vi "LaneExtractorHenesUseNetwork.vi"() -> ()   [LabVIEW 2024]
uses:
  <vilib>/userDefined/High Color/IMAQdx.ctl
  System.Windows.Forms
  <vilib>/Instr/_visa.llb/VISA Set IO Buffer Mask.ctl
  <vilib>/Instr/_visa.llb/VISA Flush IO Buffer Mask.ctl
  <vilib>/Instr/_visa.llb/VISA Configure Serial Port (Instr).vi
  <vilib>/vision/driver/NI_Vision_Acquisition_Software.lvlib
panel:
  in  "Current_image":refnum<k24>(container)
  in  "Right_lane":refnum<k24>(container)
  in  "Left_lane":refnum<k24>(container)
  out "error out 5":errorcluster
  out "inference time":string="imagedecode_time: 0 ms, inference_time: 10 ms, image_save_time: 0 ms, lane_determine_time: 4 ms, debug_image_save_time: 2 ms, calculation_time: 2 ms, stanley_time: 0 ms, debug_image2_save_time: 6 ms, both"
  out "error out 3":errorcluster
  out "Image_String":string
  in  "File Path":path=path "C:/Users/JungiHong/OneDrive/Hongik/HI-RACE/2026-01/platform_1_5/ExperimentModules/LaneTracking/forTrainImages/frame_014.jpg"
  in  "UseVideo":bool
  in  "Cam No.":T1="cam0"
  in  "input_spd":i16
  in  "HENES":refnum<visa-resource-name>="COM5"
  out "E-STOP":bool
  out "Remote_M/A":bool
  out "Steer_Feed":dbl
  out "Alive_PCU":u8(slide) scale=0.0..254.0
  out "Gear_Feed":u8
  out "Speed_Feed(RPM)":dbl format="%#_g rpm"
  out "버퍼 읽기":string
  out "Speed_Feed(m/s)":dbl
  in  "HLV_Gear":u8
  in  "HLV_A/M":bool=TRUE
  in  "HLV_E-stop":bool
  out "HENES Loop Time":u32=20
  in  "v(Velocity)m/s":dbl=1.0
  in  "k(Gain)":dbl=1.0
  out "δ(OutputSteer)degrees":dbl=3.398135469980901
  out "changearray":u32=4
  out "CV Loop Time":u32=103
  in  "stop":bool
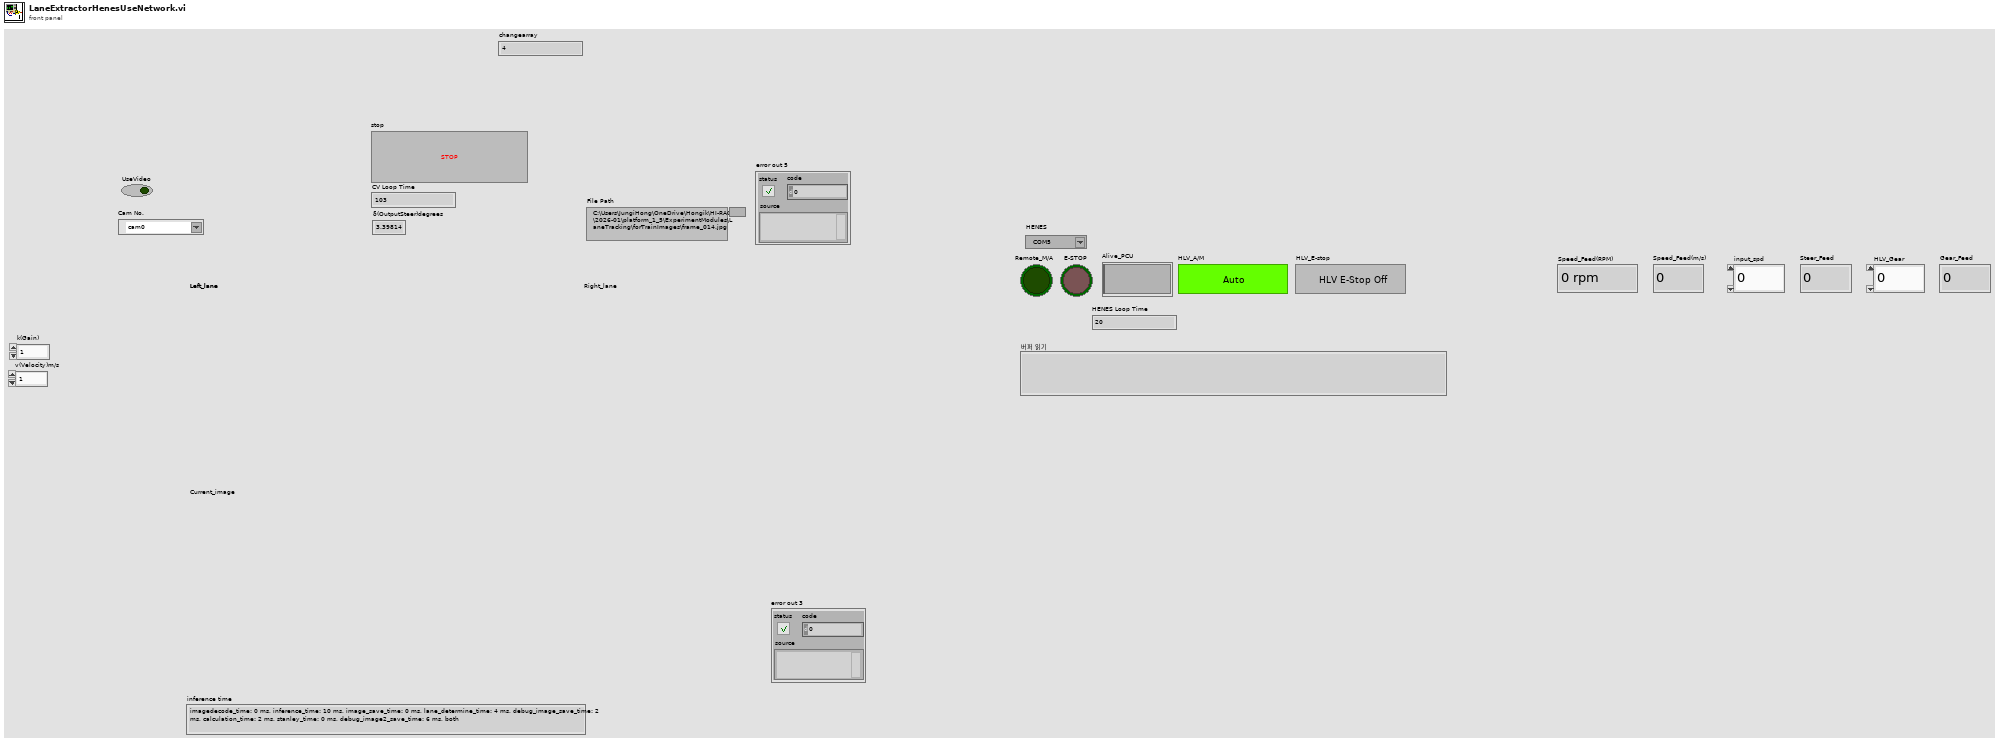
[diagram p1: front panel]
types:
  T1 = typedef "IMAQdx.ctl" = refnum<k21>
  T2 = cluster{"HENES_M/A":u8, "HENES_E-Stop":u8, "HENES_Gear":u8, "HENES_Speed":i16, "HENES_Steer":i16, "HENES_Alive":u8}
  T3 = typedef "VISA Flush IO Buffer Mask.ctl" = u16
  T4 = typedef "VISA Set IO Buffer Mask.ctl" = u16
  T5 = cluster{"HLV_M/A_Status":u8, "HLV_E-Stop":u8, "HLV_Gear":u8, "HLV_Speed":i16, "HLV_Steer":i16, "HLV_Alive":u8}
  T6 = typedef "IMAQ Image.ctl" = refnum<image>
  T7 = cluster{"Global Rectangle":i32[], "Contours":cluster{"ID":enum32{"External", "Internal"}, "Type":u32, "Coordinates":i32[]}[]}
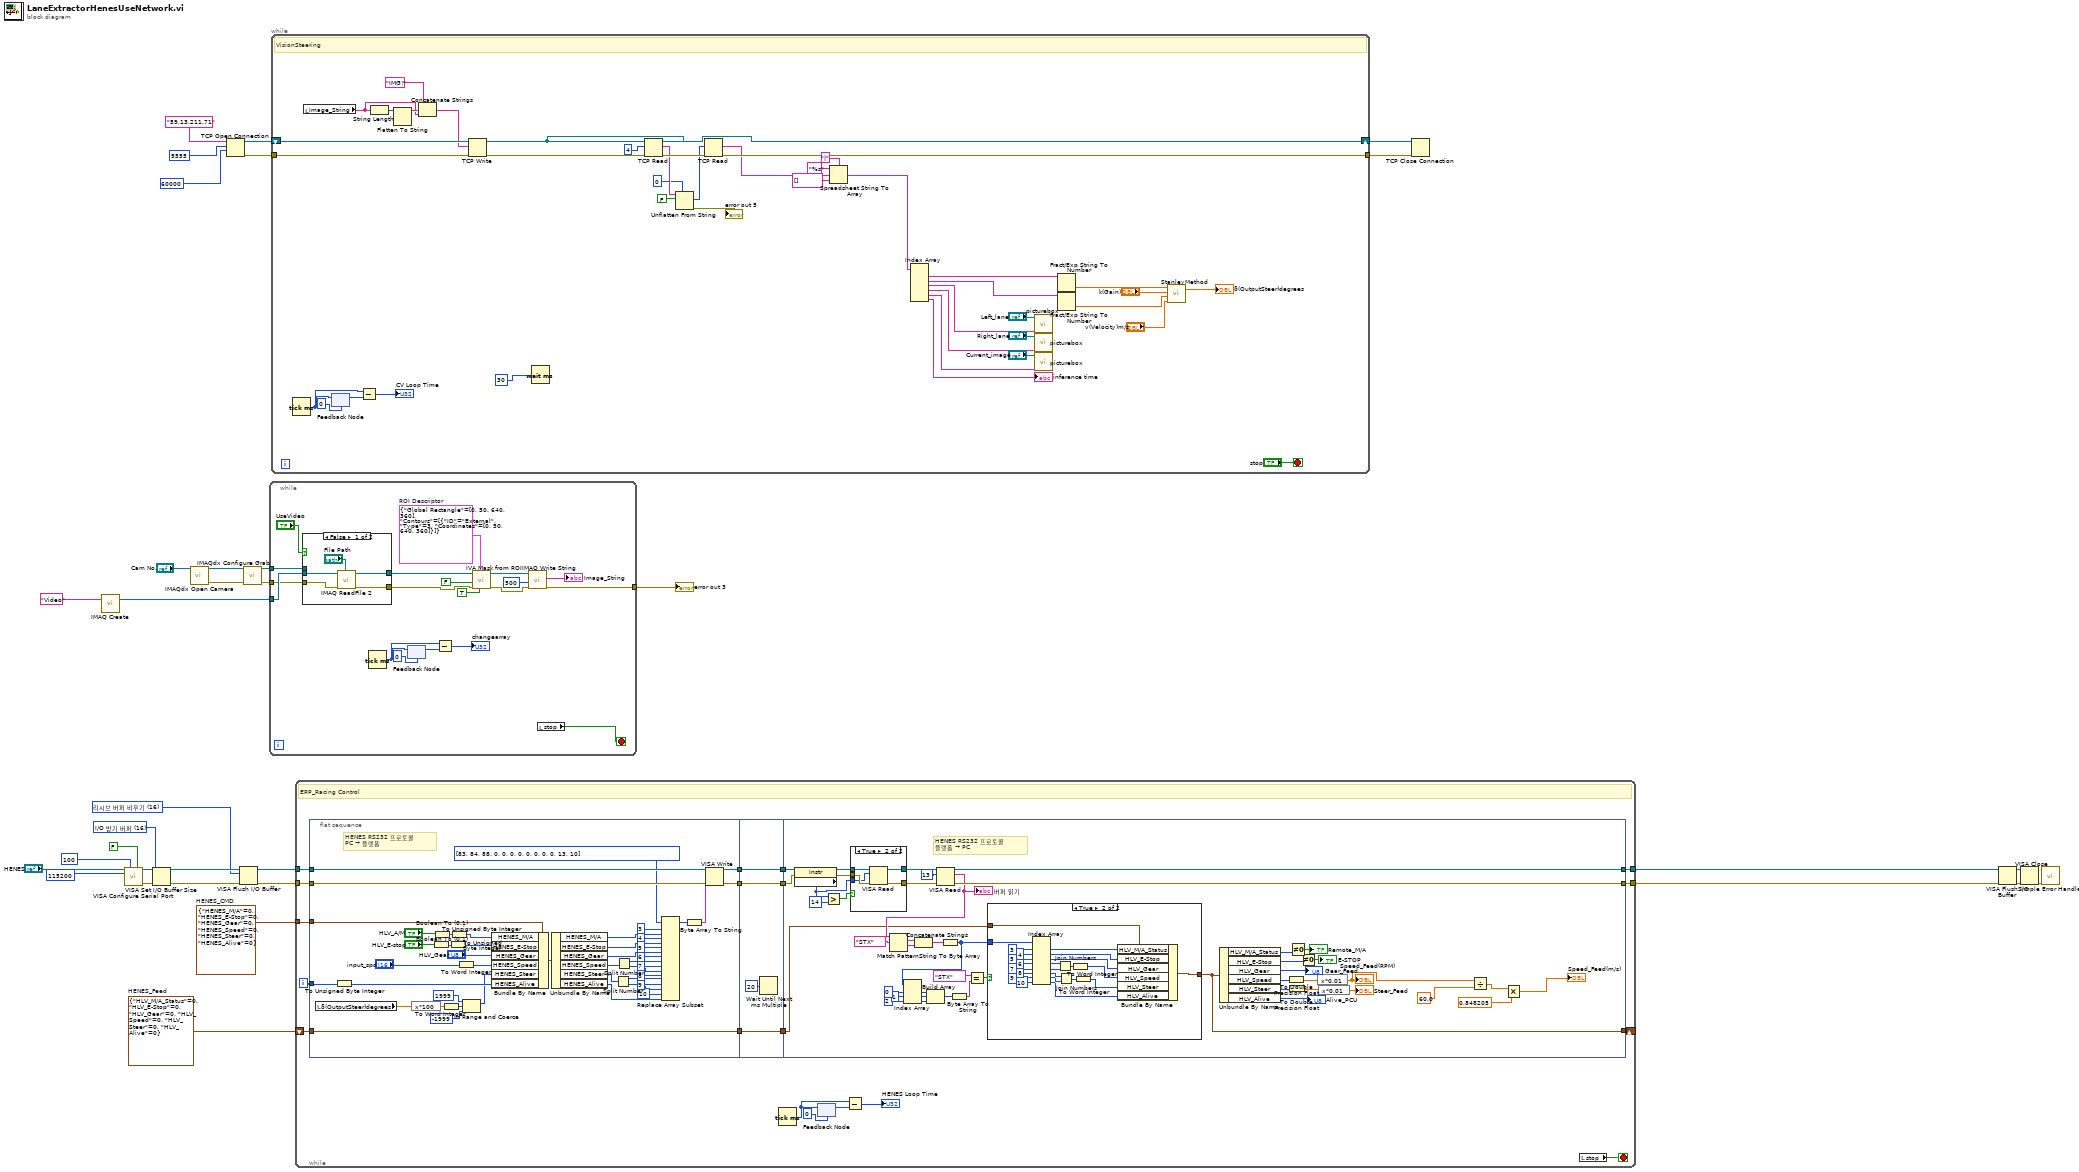
[diagram p0: block diagram]
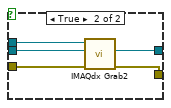
[diagram p4: hidden frame]
diagram:
  w15 = T2 {"HENES_M/A"=0, "HENES_E-Stop"=0, "HENES_Gear"=0, "HENES_Speed"=0, "HENES_Steer"=0, "HENES_Alive"=0}  # HENES_CMD
  w18 = T3 16 items=["리시브 버퍼 비우기"=16, "전달 버퍼 디바이스에 쓰기"=32, "리시브 버퍼 비우기(I/O 없음)"=64, "전달 버퍼 비우기"=128] ("Mask")
  w21 = T4 16 items=["I/O 받기 버퍼"=16, "I/O 전달 버퍼"=32, "I/O 받기와 전달 버퍼"=48] ("Mask")
  w25 = T5 {"HLV_M/A_Status"=0, "HLV_E-Stop"=0, "HLV_Gear"=0, "HLV_Speed"=0, "HLV_Steer"=0, "HLV_Alive"=0}  # HENES_Feed
  n1 = call "IMAQ Create"("Image Name"="Video") -> ("New Image"=w33:T6)  [unwired: 4 in, 1 out]
  n2 = call-poly "VISA Configure Serial Port"("VISA resource name"="HENES", "timeout (10sec)"=u32 100, "Enable Termination\nChar (T)"=FALSE ("Enable Termination\nChar (T)"), "baud rate (9600)"=u32 115200) -> ("VISA resource name out"=w17:refnum<visa-resource-name>, "error out"=w16:errorcluster)  [unwired: 10 in]
  n3 = VISA Set I/O Buffer Size(VISA resource name=w17, mask (16)=w21, error in (no error)=w16) -> (VISA resource name out=w20:refnum<visa-resource-name>, error out=w19:errorcluster)  [unwired: 1 in]
  n4 = call <vilib>:"IMAQdx Open Camera.vi"("Session In"="Cam No.") -> ("error out"=w11:errorcluster, "Session Out"=w12:T1)  [unwired: 9 in]
  n5 = TCP Open Connection(address="59.13.211.71", remote port or service name=u16 5555, timeout ms (60000)=60000) -> (connection ID=w3:refnum<k5>, error out=w4:errorcluster)  [unwired: 2 in]
  n6 = VISA Flush I/O Buffer(VISA resource name=w20, mask (16)=w18, error in (no error)=w19) -> (VISA resource name out=w30:refnum<visa-resource-name>, error out=w29:errorcluster)
  n7 = call <vilib>:"IMAQdx Configure Grab.vi"("error in"=w11, "Session In"=w12) -> ("error out"=w10:errorcluster, "Session Out"=w13:T1)  [unwired: 8 in]
  n8 = while {
    tunnel: w33 -> [w48]
    tunnel: w13 -> [w47]
    tunnel: w10 -> [w46]
    tunnel: [w38] -> w8
    stop <- w53 stop-if-true
    w43 = T7 {"Global Rectangle"=[0, 50, 640, 360], "Contours"=[{"ID"=enum."External", "Type"=3, "Coordinates"=[0, 50, 640, 360]}]}  # ROI Descriptor
    n9 = case shown="False" "UseVideo" {
      tunnel: w48 -> [w56 w63]
      tunnel: [w58 w62] -> w36
      tunnel: [w57 w61] -> w41
      tunnel: w47 -> [_ w60]
      tunnel: w46 -> [w54 w59]
      frame False {
        n10 = call "IMAQ ReadFile 2"("File Path"="File Path", "error in (no error)"=w54, "Image"=w56) -> ("error out"=w58:errorcluster, "Image Out"=w57:T6)  [unwired: 4 in, 3 out]
      }
      frame True {
        n11 = call <vilib>:"IMAQdx Grab2.vi"("error in"=w59, "Image In"=w63, "Session In"=w60) -> ("error out"=w62:errorcluster, "Image Out"=w61:T6)  [unwired: 5 in, 2 out]
      }
    }
    n12 = Tick Count (ms)() -> (millisecond timer value=w49:u32)
    n13 = feedback #1(u32 0 ("millisecond timer value")) -> (w50:u32)
    n14 = feedback-in #1(w49) -> ()
    n15 = Subtract(x=w49, y=w50) -> (x-y=→"changearray":u32)
    n16 = call <vilib>:"IVA Mask from ROI.vi"("Shrink"=TRUE, "ROI Descriptor"=w43, "error in (no error)"=w36, "Out / In"=FALSE, "Image Src"=w41) -> ("error out"=w35:errorcluster, "Image Out"=w39:T6)  [unwired: 5 out]
    n17 = call-poly "IMAQ Write String"("error in (no error)"=w35, "Image Quality"=u32 500, "Image"=w39) -> ("error out"=w38:errorcluster, "FileString"=→"Image_String":string)  [unwired: 6 in, 1 out]
    n18 = local read "stop"() -> (w53:bool)
  }
  "error out 3" <- w8
  n19 = while {
    tunnel: w4 -> [w77]
    tunnel: [w89] -> w2
    shift-right: [w87] -> w1
    shift-left: w3 -> [w78]
    stop <- "stop" stop-if-true
    # "VisionSteering"
    n20 = Tick Count (ms)() -> (millisecond timer value=w105:u32)
    n21 = local read "Image_String"() -> (w72:string)
    n22 = feedback #2(u32 0 ("millisecond timer value")) -> (w104:u32)
    n23 = feedback-in #2(w105) -> ()
    n24 = Subtract(x=w105, y=w104) -> (x-y=→"CV Loop Time":u32)
    n25 = String Length(string=w72) -> (length=w74:i32)
    n26 = Flatten To String(anything=w74) -> (data string=w73:string)  [unwired: 3 in, 2 out]
    n27 = Concatenate Strings("IMG!" ("Image_String"), w73, w72) -> (w70:string)
    n28 = TCP Write(connection ID=w78, data in=w70, error in (no error)=w77) -> (connection ID out=w79:refnum<k5>, error out=w80:errorcluster)  [unwired: 1 in, 1 out]
    n29 = Wait (ms)(milliseconds to wait=u32 30) -> ()  [unwired: 1 out]
    n30 = TCP Read(connection ID=w79, bytes to read=4, error in (no error)=w80) -> (connection ID out=w87:refnum<k5>, data out=w84:string, error out=w86:errorcluster)  [unwired: 2 in]
    n31 = Unflatten From String(type=u32 0 ("CV Loop Time 2"), binary string=w84, data includes array or string size? (T)=FALSE) -> (value=w85:u32, error out=→"error out 5":errorcluster)  [unwired: 2 in, 1 out]
    n32 = TCP Read(connection ID=w79, bytes to read=w85, error in (no error)=w86) -> (data out=w88:string, error out=w89:errorcluster)  [unwired: 2 in, 1 out]
    n33 = Spreadsheet String To Array(delimiter (Tab)="|", format string="%s", spreadsheet string=w88, array type (2D Dbl)=string[] []) -> (array=w90:string[])
    n34 = Index Array(array=w90) -> (element #1=w93:string, element #2=w92:string, element #3=w69:string, element #4=w65:string, element #5=w64:string, element #6=→"inference time":string)  [unwired: 6 in]
    n35 = call "picturebox.vi"("s"=w69, "PictureBox"="Left_lane") -> ()  [unwired: 10 in]
    n36 = call "picturebox.vi"("s"=w65, "PictureBox"="Right_lane") -> ()  [unwired: 10 in]
    n37 = call "picturebox.vi"("s"=w64, "PictureBox"="Current_image") -> ()  [unwired: 10 in]
    n38 = Fract/Exp String To Number(string=w93) -> (number=w100:dbl)  [unwired: 3 in, 1 out]
    n39 = Fract/Exp String To Number(string=w92) -> (number=w99:dbl)  [unwired: 3 in, 1 out]
    n40 = call "StanleyMethod.vi"("v(Velocity)m/s"="v(Velocity)m/s", "e(Cross-Track Err)m/s"=w99, "k(Gain)"="k(Gain)", "ψ(Heading Err)radian"=w100) -> ("δ(OutputSteer)degrees"=→"δ(OutputSteer)degrees":dbl)  [unwired: 1 out]
  }
  n41 = while {
    tunnel: w30 -> [w125]
    tunnel: w29 -> [w124]
    tunnel: [w118] -> w28
    tunnel: [w117] -> w27
    shift-right: [w112] -> _
    shift-left: w25 -> [w115]
    tunnel: w15 -> [w113]
    i -> [w119]
    stop <- w107 stop-if-true
    # "ERP_Racing Control"
    n42 = flat-sequence {
      tunnel: [w168] -> w122
      tunnel: [w167] -> w120
      tunnel: w125 -> [w170]
      tunnel: w124 -> [w169]
      tunnel: w119 -> [w166]
      tunnel: [w165] -> w116
      tunnel: w115 -> [w165]
      tunnel: w113 -> [w164]
      tunnel: [w174] -> w123
      tunnel: w122 -> [w174]
      tunnel: [w173] -> w121
      tunnel: w120 -> [w173]
      tunnel: w116 -> [w171]
      tunnel: [w171] -> w114
      tunnel: w123 -> [w202]
      tunnel: w121 -> [w201]
      tunnel: [w219] -> w118
      tunnel: [w218] -> w117
      tunnel: w114 -> [w193]
      tunnel: [w191] -> w112
      frame #0 {
        # "HENES RS232 프로토콜\nPC → 플랫폼"
        n43 = local read "δ(OutputSteer)degrees"() -> (w126:dbl)
        n44 = To Unsigned Byte Integer(number=w166) -> (unsigned 8bit integer=w153:u8)
        n45 = expression code="x*100"(w126) -> (w128:dbl)
        n46 = Boolean To (0,1)(Boolean="HLV_E-stop") -> (0, 1=w148:i16)
        n47 = Boolean To (0,1)(Boolean="HLV_A/M") -> (0, 1=w149:i16)
        n48 = To Word Integer(number=w128) -> (16bit integer=w131:i16)
        n49 = To Unsigned Byte Integer(number=w148) -> (unsigned 8bit integer=w146:u8)
        n50 = To Unsigned Byte Integer(number=w149) -> (unsigned 8bit integer=w147:u8)
        n51 = To Word Integer(number="input_spd") -> (16bit integer=w140:i16)
        n52 = In Range and Coerce(upper limit=i16 1999 ("상위 리미트"), x=w131, lower limit=i16 -1999 ("상위 리미트")) -> (coerced(x)=w139:i16)  [unwired: 1 out]
        n53 = Bundle By Name(cluster=w164, "HENES_M/A"=w147, "HENES_E-Stop"=w146, "HENES_Gear"="HLV_Gear", "HENES_Speed"=w140, "HENES_Steer"=w139, "HENES_Alive"=w153) -> (w157:T2)
        n54 = Unbundle By Name(w157) -> ("HENES_M/A"=w143:u8, "HENES_E-Stop"=w142:u8, "HENES_Gear"=w132:u8, "HENES_Speed"=w135:i16, "HENES_Steer"=w138:i16, "HENES_Alive"=w152:u8)
        n55 = Split Number(x=w138) -> (hi(x)=w137:u8, lo(x)=w136:u8)
        n56 = Split Number(x=w135) -> (hi(x)=w134:u8, lo(x)=w133:u8)
        n57 = Replace Array Subset(array=u8[] [83, 84, 88, 0, 0, 0, 0, 0, 0, 0, 0, 13, 10] ("unsigned byte array"), new element #1=w143, index #1=3, new element #2=w142, index #2=4, new element #3=w132, index #3=5, new element #4=w134, index #4=6, new element #5=w133, index #5=7, new element #6=w137, index #6=8, new element #7=w136, index #7=9, new element #8=w152, index #8=10) -> (w155:u8[])
        n58 = Byte Array To String(unsigned byte array=w155) -> (string=w154:string)
        n59 = VISA Write(VISA resource name=w170, write buffer=w154, error in (no error)=w169) -> (VISA resource name out=w168:refnum<visa-resource-name>, error out=w167:errorcluster)  [unwired: 1 out]
      }
      frame #1 {
        n60 = Wait Until Next ms Multiple(millisecond multiple=u32 20 ("대기 시간 (ms)")) -> ()  [unwired: 1 out]
      }
      frame #2 {
        # "HENES RS232 프로토콜\n플랫폼 → PC"
        n61 = property class="Instr"(reference=w202, error in=w201) -> (reference out=w182:refnum<visa-resource-name>, error out=w181:errorcluster, "Serial Settings:Number of Bytes at Serial Port"=w180:u32)
        n62 = Greater?(x=w180, y=u32 14) -> (0:w198:bool)
        n63 = case shown="True" w198 {
          tunnel: w182 -> [w246 w251]
          tunnel: w181 -> [w245 w250]
          tunnel: [w246 w249] -> w200
          tunnel: [w245 w248] -> w199
          tunnel: w180 -> [_ w247]
          frame False {
          }
          frame True {
            n64 = VISA Read(VISA resource name=w251, byte count=w247, error in (no error)=w250) -> (VISA resource name out=w249:refnum<visa-resource-name>, error out=w248:errorcluster)  [unwired: 2 out]
          }
        }
        n65 = VISA Read(VISA resource name=w200, byte count=u32 13, error in (no error)=w199) -> (VISA resource name out=w219:refnum<visa-resource-name>, read buffer=w217:string, error out=w218:errorcluster)  [unwired: 1 out]
        "버퍼 읽기" <- w217
        n66 = Match Pattern(string=w217, regular expression="STX") -> (match substring=w214:string, after substring=w215:string)  [unwired: 1 in, 2 out]
        n67 = Concatenate Strings(w214, w215) -> (w213:string)
        n68 = String To Byte Array(string=w213) -> (unsigned byte array=w195:u8[])
        n69 = Index Array(array=w195, index #1=0, index #2=1, index #3=2) -> (element #1=w208:u8, element #2=w207:u8, element #3=w206:u8)
        n70 = Build Array(w208, w207, w206) -> (w205:u8[])
        n71 = Byte Array To String(unsigned byte array=w205) -> (string=w203:string)
        n72 = Equal?(x="STX", y=w203) -> (x = y?=w194:bool)
        n73 = case shown="True" w194 {
          tunnel: w195 -> [_ w244]
          tunnel: [w221 w231] -> w191
          tunnel: w193 -> [w221 w233]
          frame False {
          }
          frame True {
            n74 = Index Array(array=w244, index #1=3, index #2=4, index #3=5, index #4=6, index #5=7, index #6=8, index #7=9, index #8=10) -> (element #1=w232:u8, element #2=w230:u8, element #3=w229:u8, element #4=w228:u8, element #5=w227:u8, element #6=w225:u8, element #7=w224:u8, element #8=w222:u8)
            n75 = Join Numbers(hi=w228, lo=w227) -> ((hi.lo)=w235:u16)
            n76 = Join Numbers(hi=w225, lo=w224) -> ((hi.lo)=w234:u16)
            n77 = To Word Integer(number=w235) -> (16bit integer=w226:i16)
            n78 = To Word Integer(number=w234) -> (16bit integer=w223:i16)
            n79 = Bundle By Name(cluster=w233, "HLV_M/A_Status"=w232, "HLV_E-Stop"=w230, "HLV_Gear"=w229, "HLV_Speed"=w226, "HLV_Steer"=w223, "HLV_Alive"=w222) -> (w231:T5)
          }
        }
        n80 = Unbundle By Name(w191) -> ("HLV_M/A_Status"=w192:u8, "HLV_E-Stop"=w186:u8, "HLV_Gear"=→"Gear_Feed":u8, "HLV_Speed"=w184:i16, "HLV_Steer"=w183:i16, "HLV_Alive"=→"Alive_PCU":u8)
        n81 = To Double Precision Float(number=w184) -> (double precision float=w196:dbl)
        n82 = To Double Precision Float(number=w183) -> (double precision float=w189:dbl)
        n83 = Not Equal To 0?(x=w192) -> (x != 0?=→"Remote_M/A":bool)
        n84 = Not Equal To 0?(x=w186) -> (x != 0?=→"E-STOP":bool)
        n85 = expression code="x*0.01"(w196) -> (w175:dbl)
        "Speed_Feed(RPM)" <- w175
        n86 = expression code="x*0.01"(w189) -> (→"Steer_Feed":dbl)
        n87 = Divide(x=w175, y=60.0) -> (x/y=w179:dbl)
        n88 = Multiply(x=w179, y=0.848205) -> (x*y=→"Speed_Feed(m/s)":dbl)
      }
    }
    n89 = Tick Count (ms)() -> (millisecond timer value=w109:u32)
    n90 = feedback #3(u32 0 ("millisecond timer value")) -> (w110:u32)
    n91 = feedback-in #3(w109) -> ()
    n92 = Subtract(x=w109, y=w110) -> (x-y=→"HENES Loop Time":u32)
    n93 = local read "stop"() -> (w107:bool)
  }
  n94 = TCP Close Connection(connection ID=w1, error in (no error)=w2) -> ()  [unwired: 1 in, 2 out]
  n95 = VISA Flush I/O Buffer(VISA resource name=w28, error in (no error)=w27) -> (VISA resource name out=w31:refnum<visa-resource-name>, error out=w32:errorcluster)  [unwired: 1 in]
  n96 = VISA Close(VISA resource name=w31, error in (no error)=w32) -> (error out=w26:errorcluster)
  n97 = call <vilib>:"Simple Error Handler.vi"("error in (no error)"=w26) -> ()  [unwired: 4 in, 5 out]
